vi "Initialize.vi"(8 "error in":errorcluster, 10 "parameters":variant, 11 "StepNode in":refnum<class "StepNode.lvclass">) -> (0 "error out":errorcluster, 2 "summary":T2[](array[typedef]), 3 "data value reference":T1)   [LabVIEW 2015, in "StepNode.lvclass"]
doc: "Initializes the data of a node to its default state.\nThe object is not created inside of this VI, because it is created from a File depending on user selection.\nCopyright 2017 National Instruments Corporation\n\nLicensed under the Apache License, Version 2.0 (the \"License\"); you may not use this file except in compliance with the License. You may obtain a copy of the License at http://www.apache.org/licenses/LICENSE-2.0\nUnless required by applicable law or agreed to in writing, software distributed under the License is distributed on an \"AS IS\" BASIS, WITHOUT WARRANTIES OR CONDITIONS OF ANY KIND, either express or implied. See the License for the specific language governing permissions and limitations under the License."
uses:
  StepNode.lvclass
  <vilib>/NI/Configuration Framework/Node/Summary.ctl
  <vilib>/NI/Configuration Framework/Node/NodeRef.ctl
  <vilib>/NI/Configuration Framework/Node/NISE_CEF_Node.lvclass
  Prototype/classes/Step/Config/Step Config.lvclass
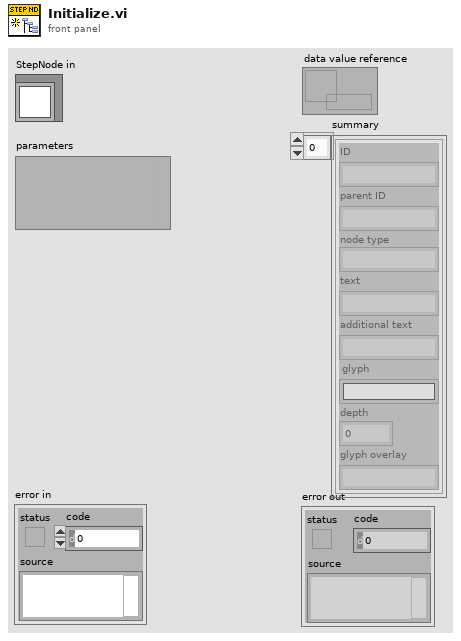
[diagram p1: front panel]
types:
  T1 = typedef "NISE_CEF_Node.lvclass/NodeRef.ctl" = refnum<data-value>
  T2 = typedef "NISE_CEF_Node.lvclass/Summary.ctl" = cluster{"ID":string, "parent ID":string, "node type":string, "text":string, "additional text":string, "glyph":string, "depth":i32, "glyph overlay":string}
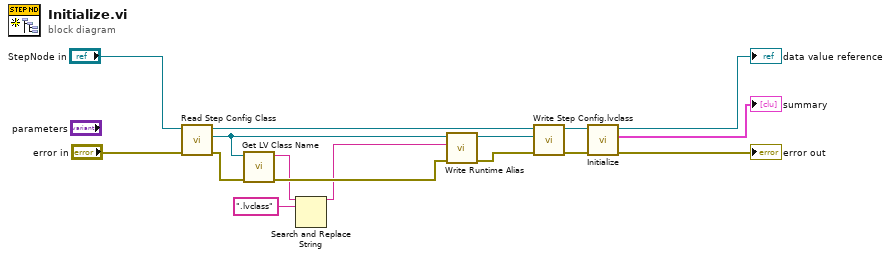
[diagram p0: block diagram]
diagram:
  n1 = call-dynamic "Read Step Config Class.vi"("error in (no error)"="error in", "StepNode in"="StepNode in") -> ("error out"=w12:errorcluster, "Step Config.lvclass"=w5:refnum<class "Step Config.lvclass">, "StepNode out"=w10:refnum<class "StepNode.lvclass">)  [unwired: 7 in]
  n2 = call <vilib>:"Get LV Class Name.vi"("error in (no error)"=w12, "object"=w5) -> ("error out"=w6:errorcluster, "class name"=w4:string)  [unwired: 8 in]
  n3 = Search and Replace String(input string=w4, search string=".lvclass") -> (result string=w2:string)  [unwired: 6 in, 3 out]
  n4 = call-dynamic "Write Runtime Alias.vi"("error in (no error)"=w6, "Runtime Alias"=w2, "Step Config in"=w5) -> ("error out"=w8:errorcluster, "Step Config out"=w7:refnum<class "Step Config.lvclass">)  [unwired: 7 in]
  n5 = call-dynamic "Write Step Config.lvclass.vi"("error in (no error)"=w8, "Step Config.lvclass"=w7, "StepNode in"=w10) -> ("error out"=w11:errorcluster, "StepNode out"=w9:refnum<class "StepNode.lvclass">)  [unwired: 7 in]
  n6 = call-parent "Initialize.vi"("error in"=w11, "node in"=w9) -> ("error out"=→"error out":errorcluster, "summary"=→"summary":T2[], "data value reference"=→"data value reference":T1)  [unwired: 7 in]
